vi "Delete_Password_Reset_File.vi"() -> ()   [LabVIEW 2016]
panel:
  out "error out":errorcluster
  out "cancelled":bool
  out "deleted path":path
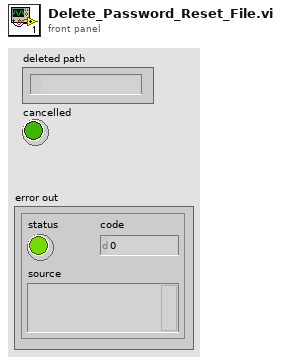
[diagram p1: front panel]
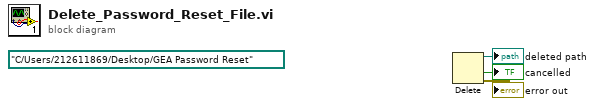
[diagram p0: block diagram]
diagram:
  (unwired) path "C:/Users/212611869/Desktop/GEA Password Reset" ("path (use dialog)")
  n1 = Delete() -> (deleted path=→"deleted path":path, cancelled=→"cancelled":bool, error out=→"error out":errorcluster)  [unwired: 5 in]
